vi "S7_StopCom.vi"(8 "错误输入":errorcluster caption="错误输入（无错误）", 11 "connect id":refnum<k24>) -> (0 "错误输出":errorcluster, 1 "IsSuccess":bool, 3 "connect id":refnum<k24>)   [LabVIEW 2018]
uses:
  E:/Fergus/S7/S7_code/Lib/HslCommunication.dll
  Lib/HslCommunication.dll
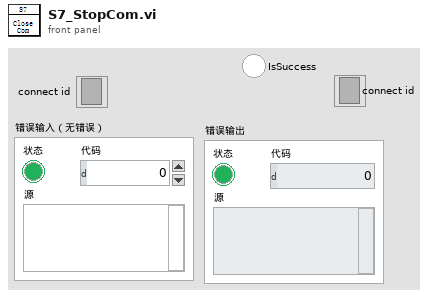
[diagram p1: front panel]
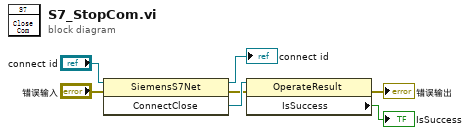
[diagram p0: block diagram]
diagram:
  n1 = invoke on="调用节点" class="SiemensS7Net" method="ConnectClose"(reference="connect id", error in="错误输入") -> (reference out=→"connect id":refnum<k24>, error out=w4:errorcluster, "ConnectClose"=w5:refnum<k24>)  [unwired: 1 in]
  n2 = property class="OperateResult"(reference=w5, error in=w4) -> (error out=→"错误输出":errorcluster, "IsSuccess"=→"IsSuccess":bool)  [unwired: 1 out]
